vi "GetCurrentLight.vi"(0 "object in":refnum<class "TrafficLight.lvclass">, 5 "Error In":errorcluster) -> (14 "object out":refnum<class "TrafficLight.lvclass">, 16 "CurrentLight":enum16{"RED", "YELLOW", "GREEN"}(ring), 19 "Error Out":errorcluster)   [LabVIEW 2024, in "TrafficLight.lvclass"]
uses:
  TrafficLight.lvclass
  TrafficLight.lvclass/TrafficLight.ctl
panel:
  # "Connector Pane"
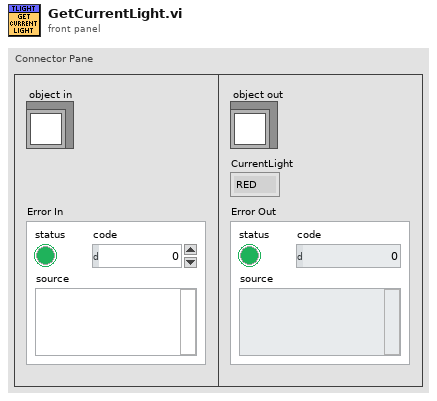
[diagram p1: front panel]
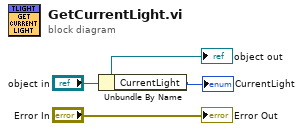
[diagram p0: block diagram]
diagram:
  n1 = Unbundle By Name("object in") -> ("CurrentLight"=→"CurrentLight":enum16{"RED", "YELLOW", "GREEN"})
  "Error Out" <- "Error In"
  "object out" <- "object in"
